vi "putNodeOnClosed.vi"(8 "error in (no error)":errorcluster, 10 "GraphNode in":refnum<data-value>, 11 "Graph in":refnum<class "Graph.lvclass">) -> (0 "error out":errorcluster, 2 "GraphNode out":refnum<data-value>, 3 "Graph out":refnum<class "Graph.lvclass">)   [LabVIEW 2010, in "Graph.lvclass"]
doc: "Puts a node on the CLOSED list. The CLOSED list is used to keep track what nodes have already been searched so that we don't search them again."
uses:
  Graph.lvclass
  GraphNode/GraphNode.lvclass
  Graph.lvclass/Graph.ctl
  LinkedList/position.ctl
  LinkedList/LinkedList.lvclass
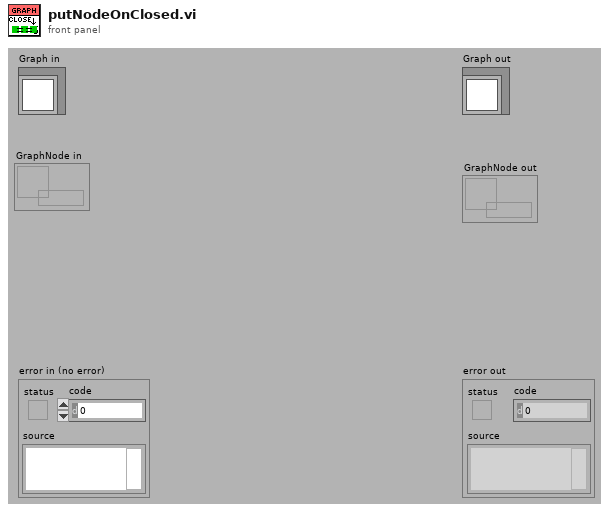
[diagram p1: front panel]
types:
  T1 = typedef "LinkedList.lvclass/position.ctl" = enum16{"Front", "Back", "Search"}
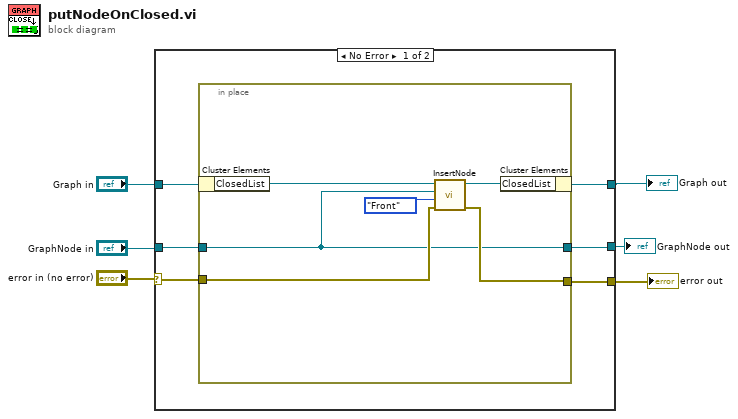
[diagram p0: block diagram]
diagram:
  n1 = case shown="No Error" "error in (no error)" {
    selector: "error in (no error)" -> [w12 w21]
    tunnel: [w10 w21] -> w3
    tunnel: [w9 w20] -> w5
    tunnel: "Graph in" -> [w11 w20]
    tunnel: "GraphNode in" -> [w8 w19]
    tunnel: [w7 w19] -> w1
    frame No Error {
      n2 = in-place {
        in-place-border: w12 -> [w14]
        in-place-border: [w16] -> w10
        in-place-border: w8 -> [w13]
        in-place-border: [w13] -> w7
        n3 = in-place-cluster #1(w11) -> ("ClosedList"=w18:refnum<class "BasicSortedList.lvclass">)
        n4 = call "InsertNode.vi"("error in (no error)"=w14, "position"=position."Front", "ToInsert"=w13, "LinkedList in"=w18) -> ("error out"=w16:errorcluster, "LinkedList out"=w17:refnum<class "BasicSortedList.lvclass">)  [unwired: 5 in, 1 out]
        n5 = in-place-cluster #1("ClosedList"=w17) -> (w9:refnum<class "Graph.lvclass">)
      }
    }
    frame Error {
    }
  }
  "error out" <- w3
  "Graph out" <- w5
  "GraphNode out" <- w1
